vi "goToPointA2.vi"() -> ()   [LabVIEW 2021, in "KickToSkill.lvclass"]
uses:
  KickToSkill.lvclass
  Robot_class/Robot.lvclass
  Game_class/Game.lvclass
  Game_class/Game.lvclass/Game.ctl
  Object_class/Object.lvclass/Object.ctl
  Robot_class/Robot.lvclass/Robot.ctl
  <vilib>/Analysis/coordinate.llb/2D Cartesian Coordinate Rotation (Scalar).vi
  Game_class/Read BallRef.vi
  Object_class/Read position(x,y).vi
  Robot_class/Write dest_x.vi
  Robot_class/Write dest_y.vi
  Robot_class/Write dest_orientation.vi
  Ball_class/Ball.lvclass
  D:/RoboIme/horie/SSL_AI/Object_class/Object.lvclass
  <vilib>/Analysis/NI_AALPro.lvlib
panel:
  out "Robot out":refnum<class "Robot.lvclass">
  in  "Raio":dbl=123.0
  in  "Game":refnum<class "Game.lvclass">
  in  "Target":dbl[](array[numeric])
  in  "Robot in":refnum<class "Robot.lvclass">
  out "KickToSkill out":refnum<class "KickToSkill.lvclass">
  in  "KickToSkill in":refnum<class "KickToSkill.lvclass">
  out "error out":errorcluster
  in  "error in (no error)":errorcluster
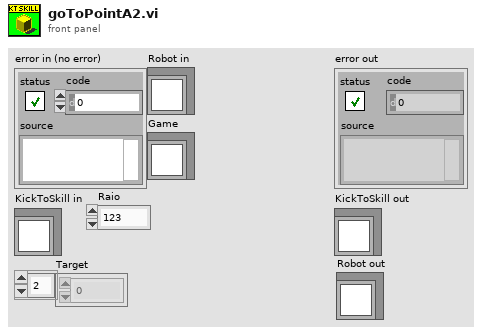
[diagram p1: front panel]
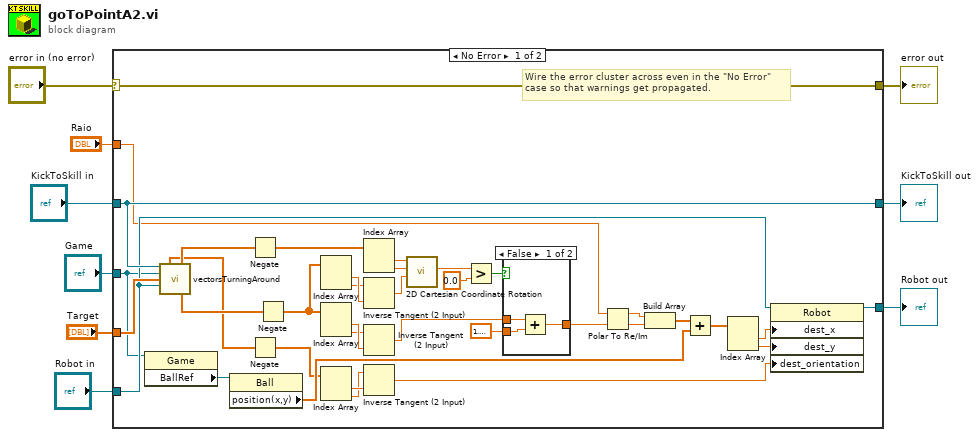
[diagram p0: block diagram]
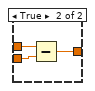
[diagram p2: hidden frame]
diagram:
  n1 = case shown="No Error" "error in (no error)" {
    selector: "error in (no error)" -> [w46 w55]
    tunnel: [w46 w55] -> w8
    tunnel: [w45 w54] -> w6
    tunnel: "KickToSkill in" -> [w45 w54]
    tunnel: "Game" -> [w25 _]
    tunnel: "Target" -> [w44 _]
    tunnel: "Robot in" -> [w42 w53]
    tunnel: [w43 w53] -> w2
    tunnel: "Raio" -> [w21 _]
    frame No Error {
      # "Wire the error cluster across even in the \"No Error\"\ncase so that warnings get propagated."
      n2 = property class="Game"(reference=w25) -> ("BallRef"=w24:refnum<class "Ball.lvclass">)  [unwired: 1 in, 2 out]
      n3 = call "vectorsTurningAround.vi"("KickToSkill in"=w45, "Game"=w25, "Target"=w44, "Robot in"=w42) -> ("Robot - Target"=w14:dbl[], "Ball - Target"=w40:dbl[], "Robot - Ball"=w36:dbl[])  [unwired: 4 in, 5 out]
      n4 = property class="Ball"(reference=w24) -> ("position(x,y)"=w15:dbl[])  [unwired: 1 in, 2 out]
      n5 = Negate(x=w40) -> (-x=w39:dbl[])
      n6 = Negate(x=w14) -> (-x=w13:dbl[])
      n7 = Negate(x=w36) -> (-x=w28:dbl[])
      n8 = Index Array(array=w28) -> (element #1=w35:dbl, element #2=w34:dbl)  [unwired: 2 in]
      n9 = Index Array(array=w28) -> (element #1=w30:dbl, element #2=w29:dbl)  [unwired: 2 in]
      n10 = Index Array(array=w13) -> (element #1=w12:dbl, element #2=w11:dbl)  [unwired: 2 in]
      n11 = Index Array(array=w39) -> (element #1=w38:dbl, element #2=w37:dbl)  [unwired: 2 in]
      n12 = Inverse Tangent (2 Input)(1:w35, 2:w34) -> (0:w41:dbl)
      n13 = Inverse Tangent (2 Input)(1:w30, 2:w29) -> (0:w27:dbl)
      n14 = Inverse Tangent (2 Input)(1:w12, 2:w11) -> (0:w10:dbl)
      n15 = call-poly <vilib>:"2D Cartesian Coordinate Rotation.vi"("theta"=w41, "y"=w37, "x"=w38) -> ("y out"=w33:dbl)  [unwired: 6 in, 2 out]
      n16 = Greater?(x=w33, y=0.0) -> (0:w31:bool)
      n17 = case shown="False" w31 {
        tunnel: w27 -> [w49 w52]
        tunnel: 1.5707963267948966 -> [w48 w51]
        tunnel: [w47 w50] -> w20
        frame False {
          n18 = Add(x=w49, y=w48) -> (x+y=w47:dbl)
        }
        frame True {
          n19 = Subtract(x=w52, y=w51) -> (x-y=w50:dbl)
        }
      }
      n20 = Polar To Re/Im(2:w20, 3:w21) -> (0:w22:dbl, 1:w23:dbl)
      n21 = Build Array(w23, w22) -> (w16:dbl[])
      n22 = Add(x=w16, y=w15) -> (x+y=w19:dbl[])
      n23 = Index Array(array=w19) -> (element #1=w18:dbl, element #2=w17:dbl)  [unwired: 2 in]
      n24 = property class="Robot"(reference=w42, "dest_x"=w18, "dest_y"=w17, "dest_orientation"=w10) -> (reference out=w43:refnum<class "Robot.lvclass">)  [unwired: 1 in, 1 out]
    }
    frame Error {
    }
  }
  "error out" <- w8
  "KickToSkill out" <- w6
  "Robot out" <- w2
